vi "Test CNV Algo and graph.vi"() -> ()   [LabVIEW 2016]
uses:
  <vilib>/Analysis/3filter.llb/Filter Passband Type.ctl
  <vilib>/Analysis/baseanly.llb/Mean (DBL).vi
  <vilib>/Utility/file.llb/Read Delimited Spreadsheet (DBL).vi
  <vilib>/Analysis/3filter.llb/Butterworth Filter (DBL).vi
  <vilib>/Analysis/NI_AALBase.lvlib
panel:
  out "index of element":i32
  out "error":i32
  out "Waveform Graph Filtered":dbl[](graph)
  out "Waveform Graph":dbl[](graph)
  out "CNV Graph":dbl[](graph)
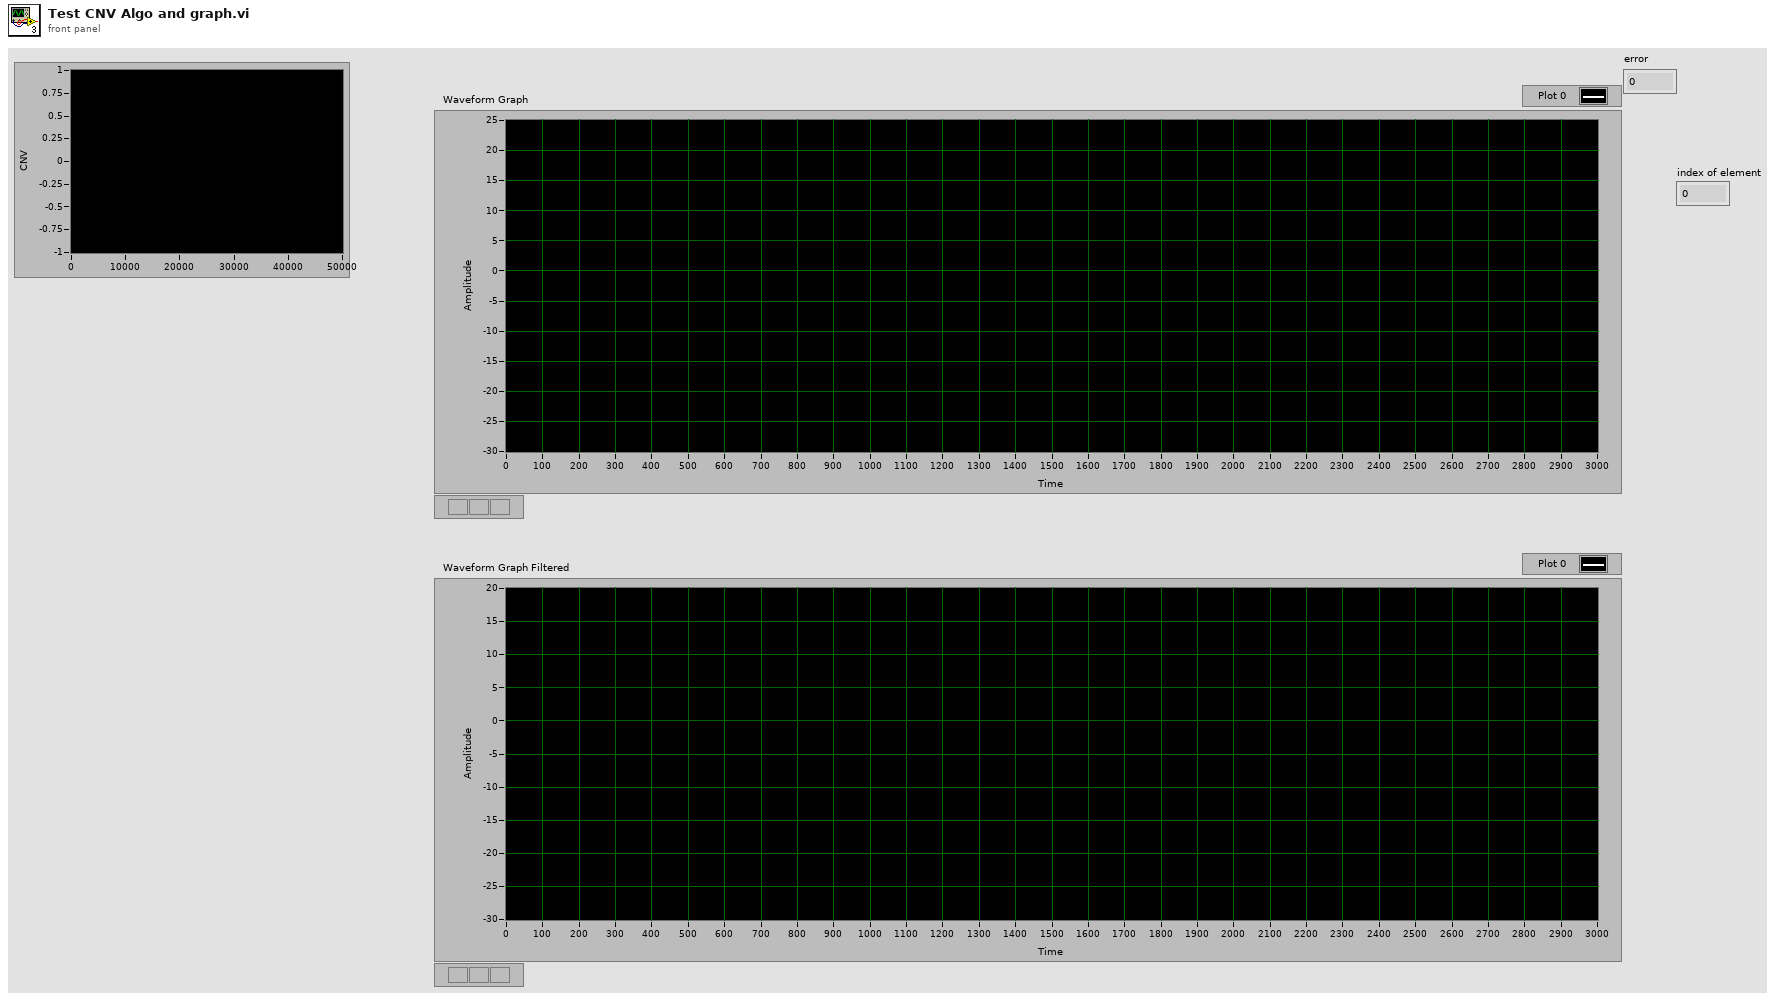
[diagram p1: front panel]
types:
  T1 = typedef "NI_AALBase.lvlib/Filter Passband Type.ctl" = enum32{"Lowpass", "Highpass", "Bandpass", "Bandstop"}
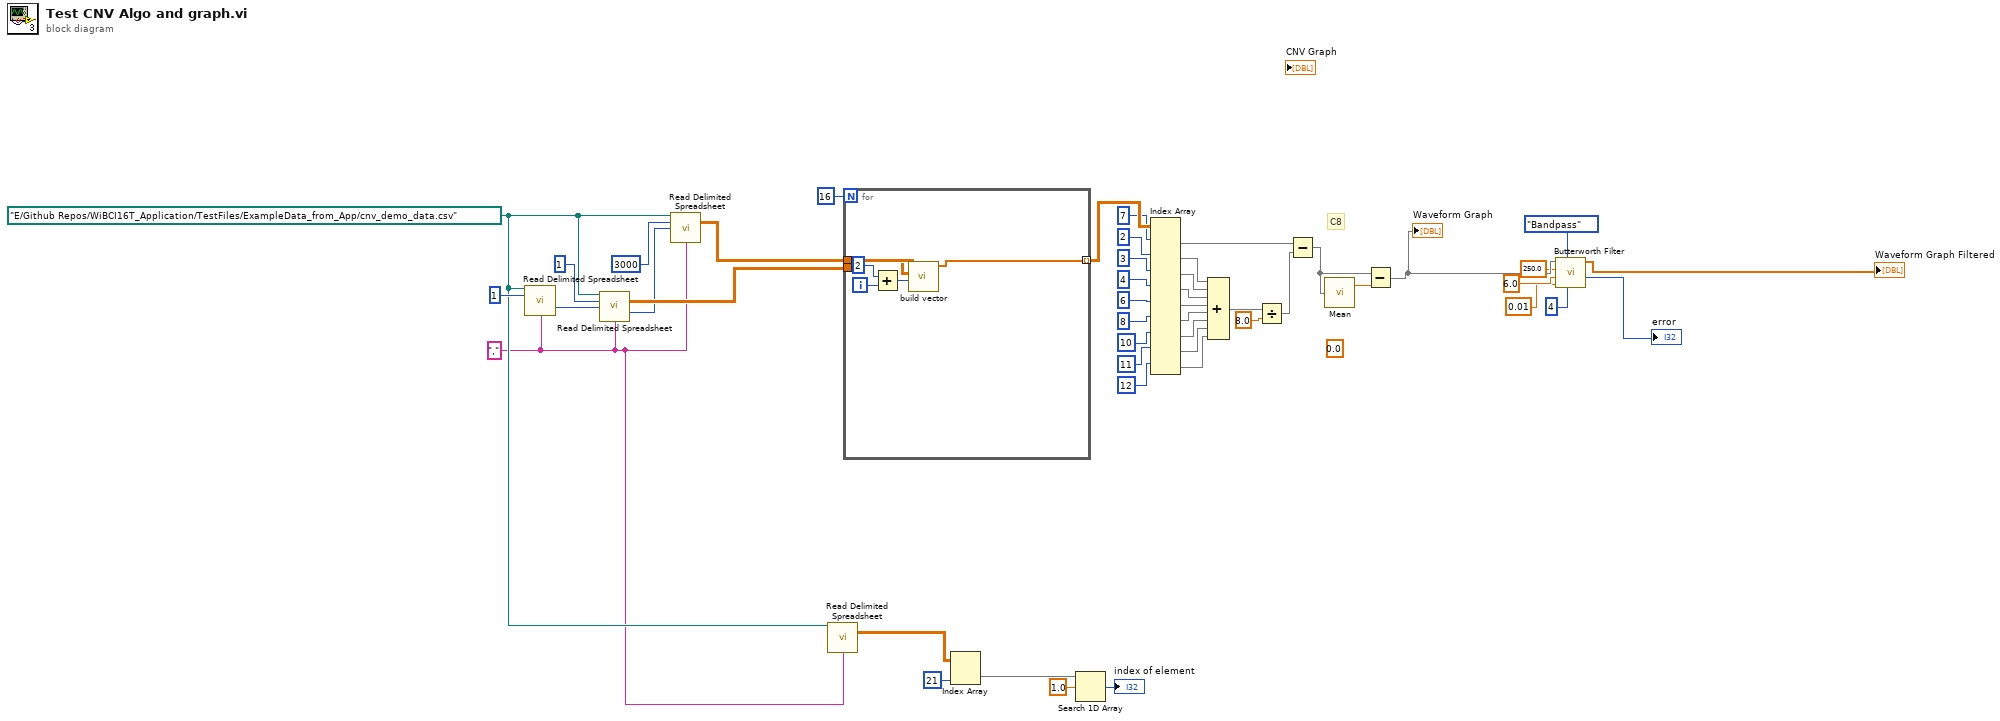
[diagram p0: block diagram]
diagram:
  (unwired) 0.0
  w5 = ","
  w6 = path "E:/Github Repos/WiBCI16T_Application/TestFiles/ExampleData_from_App/cnv_demo_data.csv" ("file path (dialog if empty)")
  # "C8"
  n1 = call-poly <vilib>:"Read Delimited Spreadsheet.vi"("file path (dialog if empty)"=w6, "number of rows (all:-1)"=1, "delimiter (\\t)"=w5) -> ("mark after read (chars.)"=w45:i32)  [unwired: 7 in, 5 out]
  n2 = call-poly <vilib>:"Read Delimited Spreadsheet.vi"("file path (dialog if empty)"=w6, "number of rows (all:-1)"=1, "start of read offset (chars.:0)"=w45, "delimiter (\\t)"=w5) -> ("all rows"=w43:dbl[][], "mark after read (chars.)"=w42:i32)  [unwired: 6 in, 4 out]
  n3 = call-poly <vilib>:"Read Delimited Spreadsheet.vi"("file path (dialog if empty)"=w6, "number of rows (all:-1)"=3000, "start of read offset (chars.:0)"=w42, "delimiter (\\t)"=w5) -> ("all rows"=w17:dbl[][])  [unwired: 6 in, 5 out]
  n4 = call-poly <vilib>:"Read Delimited Spreadsheet.vi"("file path (dialog if empty)"=w6, "delimiter (\\t)"=w5) -> ("all rows"=w4:dbl[][])  [unwired: 8 in, 5 out]
  n5 = for {
    N: 16 -> [_]
    tunnel: w17 -> [w53]
    tunnel: w43 -> [w52]
    tunnel: [w48] -> w40 mode=indexing
    i -> [w51]
    n6 = Add(x=2, y=w51) -> (x+y=w49:i32)
    n7 = call "build vector.vi"("Index"=w49, "first element"=w52, "diff data"=w53) -> ("Rebuild Vector"=w48:dbl[])  [unwired: 8 in]
  }
  n8 = Index Array(array=w4, index (col)=21 ("disabled index (col)")) -> (element=w3:dbl[])  [unwired: 1 in]
  n9 = Search 1D Array(1D array=w3, element=1.0) -> (index of element=→"index of element":i32)  [unwired: 1 in]
  n10 = Index Array(array=w40, index (row) #1=7 ("disabled index (col)"), index (row) #2=2 ("index (row)"), index (row) #3=3 ("index (row)"), index (row) #4=4 ("index (row)"), index (row) #5=6 ("index (row)"), index (row) #6=8 ("index (row)"), index (row) #7=10 ("index (row)"), index (row) #8=11 ("index (row)"), index (row) #9=12 ("index (row)")) -> (element #1=w20:dbl[], element #2=w30:dbl[], element #3=w29:dbl[], element #4=w28:dbl[], element #5=w27:dbl[], element #6=w26:dbl[], element #7=w25:dbl[], element #8=w24:dbl[], element #9=w23:dbl[])  [unwired: 9 in]
  n11 = Compound Arithmetic op=ADD(w30, w29, w28, w27, w26, w25, w24, w23) -> (w22:dbl[])
  n12 = Divide(x=w22, y=8.0) -> (x/y=w19:dbl[])
  n13 = Subtract(x=w20, y=w19) -> (x-y=w18:dbl[])
  n14 = call-poly <vilib>:"Mean.vi"("X"=w18) -> ("mean"=w15:dbl)  [unwired: 1 out]
  n15 = Subtract(x=w18, y=w15) -> (x-y=w14:dbl[])
  "Waveform Graph" <- w14
  n16 = call-poly <vilib>:"Butterworth Filter.vi"("order"=4, "filter type"=Filter_Passband_Type."Bandpass", "low cutoff freq: fl"=0.01, "high cutoff freq: fh"=6.0, "sampling freq: fs"=250.0, "X"=w14) -> ("error"=→"error":i32, "Filtered X"=→"Waveform Graph Filtered":dbl[])  [unwired: 2 in]
